vi "rs3 Advanced get HDAD3.vi"(8 "error in (no error)":errorcluster, 10 "mode":i32, 11 "device in":u64) -> (0 "error out 2":errorcluster, 1 "error":u32, 2 "HDAD":T1, 3 "Dev out":u64)   [LabVIEW 2017, in "libRealSense3.lvlib"]
doc: "Opens communication to a specific RealSense Device."
uses:
  libRealSense3.lvlib
  realsense2.dll
panel:
  # "RS3 Adv. Get HDAD 3"
  # "(C) 2017 Intel Corp.,  AGJ"
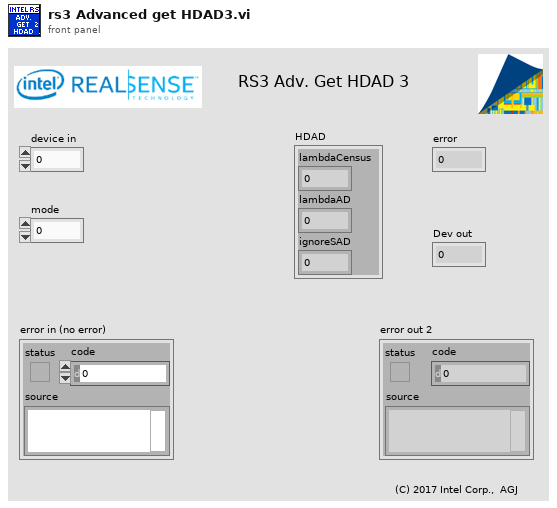
[diagram p1: front panel]
types:
  T1 = cluster{"lambdaCensus":sgl, "lambdaAD":sgl, "ignoreSAD":u32}
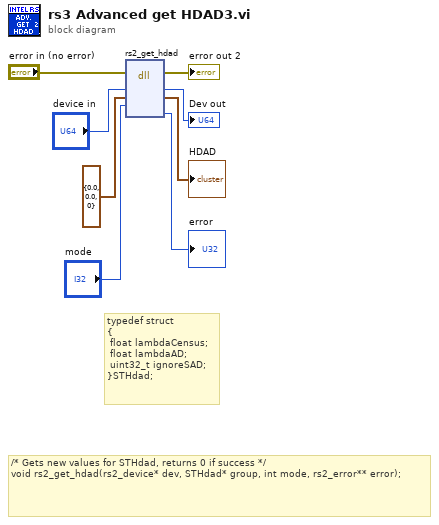
[diagram p0: block diagram]
diagram:
  # "/* Gets new values for STHdad, returns 0 if success */\nvoid rs2_get_hdad(rs2_device* dev, STHdad* group, int mode, rs2_error** error);"
  # "typedef struct\n{\n\tfloat lambdaCensus;\n\tfloat lambdaAD;\n\tuint32_t ignoreSAD;\n}STHdad;"
  n1 = dll-call lib="C:/Users/agrunnet/Documents/libRealSense6/realsense2.dll" fn="rs2_get_hdad"(error in="error in (no error)", "device"="device in", "HDAD"=T1 {"lambdaCensus"=0.0, "lambdaAD"=0.0, "ignoreSAD"=0} ("output cluster"), "mode"="mode") -> (error out=→"error out 2":errorcluster, "device"=→"Dev out":u64, "HDAD"=→"HDAD":T1, "error"=→"error":u64)  [unwired: 5 in, 1 out]
